vi "Path.vi"(1 "Relative Path":path, 2 "Base Path":path) -> (0 "Absolute Path":path)   [LabVIEW 2011]
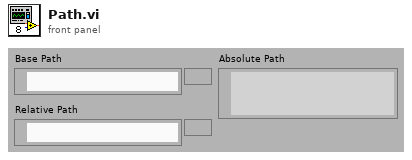
[diagram p1: front panel]
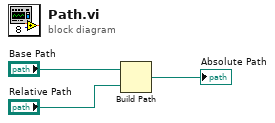
[diagram p0: block diagram]
diagram:
  n1 = Build Path(base path="Base Path", name or relative path="Relative Path") -> (appended path=→"Absolute Path":path)
